vi "Add Hardware.vi"(8 "error in (no error)":errorcluster, 10 "Hardware.lvclass":refnum<class "Hardware.lvclass">, 11 "Controller in":refnum<class "Controller.lvclass">) -> (0 "error out":errorcluster, 3 "Controller out":refnum<class "Controller.lvclass">)   [LabVIEW 2026, in "Controller Actor.lvlib" / "Controller.lvclass"]
uses:
  Controller.lvclass
  C:/Program Files/National Instruments/LabVIEW 2026/vi.lib/ActorFramework/Actor/Actor.lvclass
  Hardware/Hardware.lvclass
  Controller.lvclass/Controller.ctl
  Hardware/Hardware.lvclass/Hardware.ctl
  Extensible-Config-Dialog/Configuration.lvclass/Configuration.ctl
  <vilib>/ActorFramework/Actor/Actor.lvclass/Actor.ctl
  <vilib>/ActorFramework/Message Enqueuer/Message Enqueuer.lvclass/Message Enqueuer.ctl
  <vilib>/ActorFramework/Message Enqueuer/Init from Existing Queue.vi
  Hardware/HW Config/HW Configuration.lvclass
  C:/Users/E2013170/Documents/GitHub/Measurement-Utility-Reference/components/Extensible-Config-Dialog/Configuration.lvclass
  <vilib>/Utility/LVClass/Get LV Class Path.vi
  recovery/packages/oglib_file-4.0.1.22-8A89CE420A/File Group 0/user.lib/_OpenG.lib/file/file.llb/Strip Path Extension__ogtk.vi
  recovery/packages/oglib_file-4.0.1.22-8A89CE420A/File Group 0/user.lib/_OpenG.lib/file/file.llb/Strip Path Extension - String__ogtk.vi
  Extensible-Config-Dialog/Configuration.lvclass
  <vilib>/ActorFramework/Message Enqueuer/Message Enqueuer.lvclass
  Messages/Log Status/Log Status.lvclass
  <vilib>/ActorFramework/Actor/Actor.lvclass
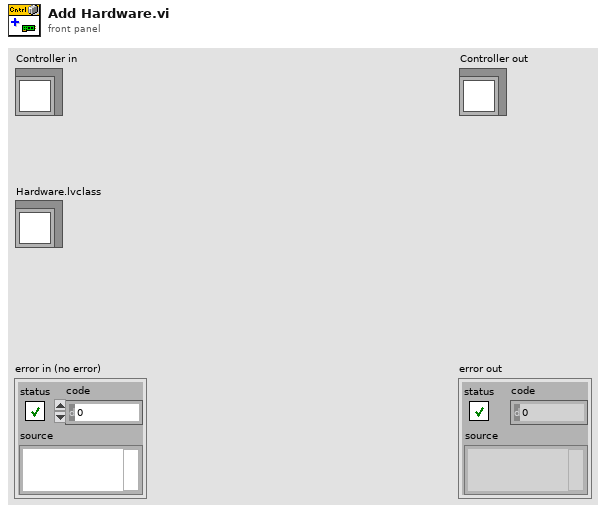
[diagram p1: front panel]
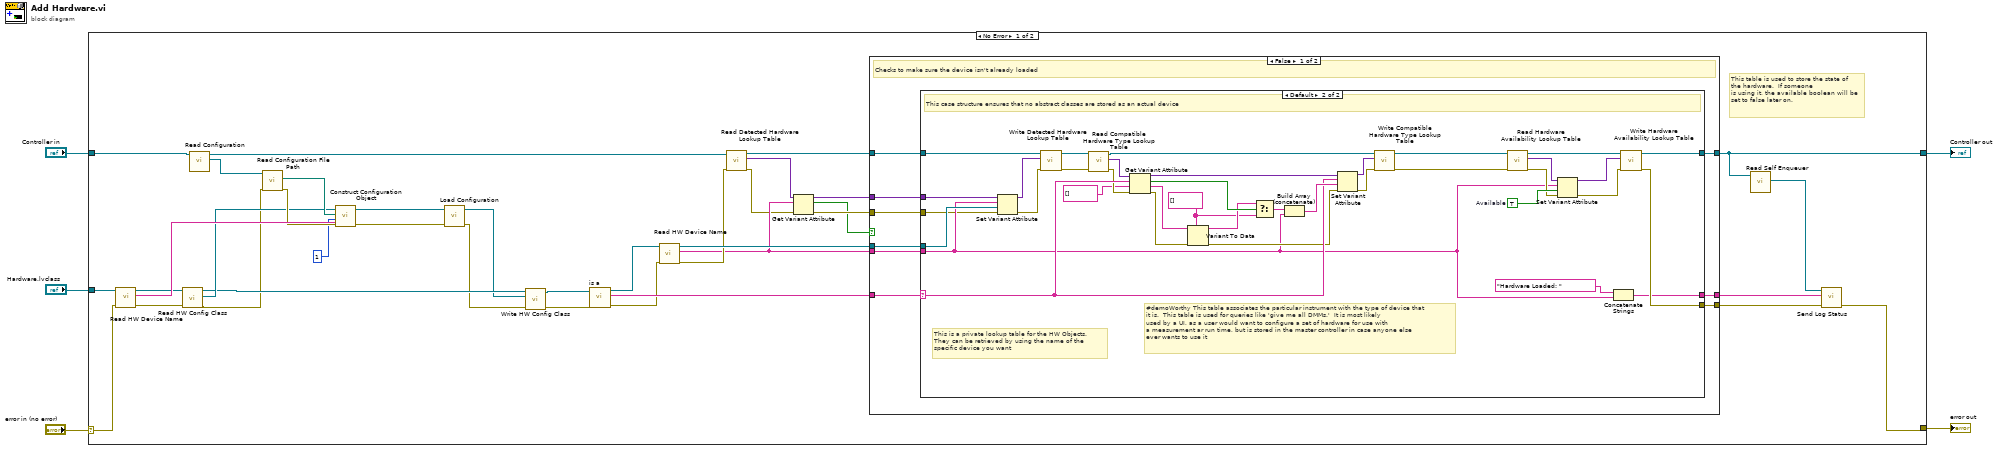
[diagram p0: block diagram]
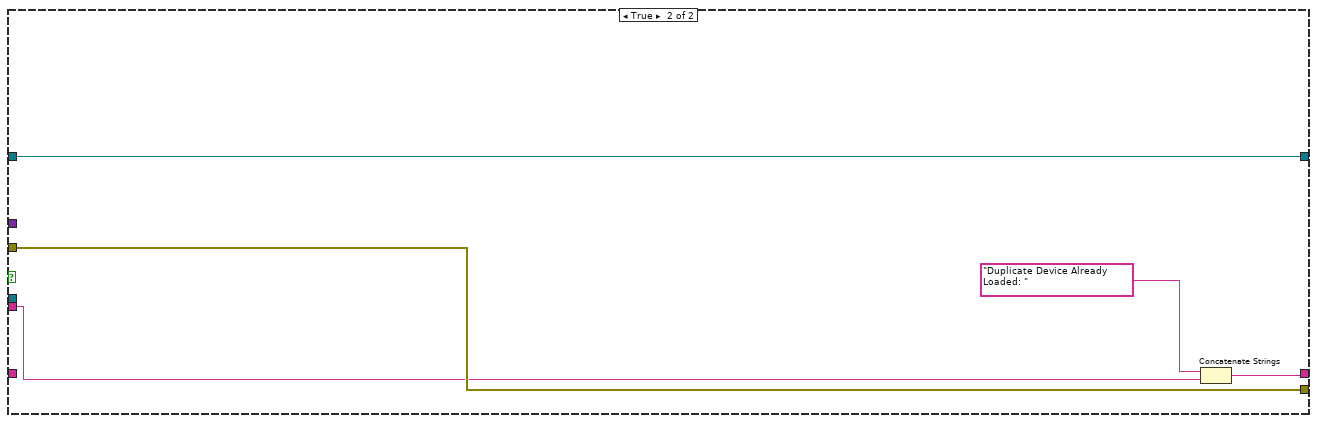
[diagram p3: hidden frame]
diagram:
  n1 = case shown="No Error" "error in (no error)" {
    selector: "error in (no error)" -> [w17 w96]
    tunnel: [w40 w96] -> w4
    tunnel: [w28 w95] -> w2
    tunnel: "Controller in" -> [w21 w95]
    tunnel: "Hardware.lvclass" -> [w19 _]
    frame No Error {
      # "This table is used to store the state of the hardware.  If someone\nis using it, the available boolean will be set to false later on."
      n2 = call "Read HW Device Name.vi"("error in (no error)"=w17, "Analog in"=w19) -> ("error out"=w13:errorcluster, "Device Name"=w18:string, "Analog out"=w14:refnum<class "Hardware.lvclass">)  [unwired: 7 in]
      n3 = call "Read HW Config Class.vi"("error in (no error)"=w13, "Hardware in"=w14) -> ("error out"=w6:errorcluster, "Hardware.lvlib:HW Configuration.lvclass"=w12:refnum<class "HW Configuration.lvclass">, "Hardware out"=w11:refnum<class "Hardware.lvclass">)  [unwired: 7 in]
      n4 = call "Read Configuration.vi"("Controller in"=w21) -> ("Configuration.lvlib:Configuration.lvclass"=w23:refnum<class "Configuration.lvclass">, "Controller out"=w20:refnum<class "Controller.lvclass">)  [unwired: 8 in, 1 out]
      n5 = call "Read Configuration File Path.vi"("error in (no error)"=w6, "Configuration in"=w23) -> ("error out"=w16:errorcluster, "Configuration File Path"=w22:path)  [unwired: 7 in, 1 out]
      n6 = call "Construct Configuration Object.vi"("Group Name"=w18, "error in (no error)"=w16, "Initial Category Selection"=1, "Configuration File Path"=w22, "Configuration in"=w12) -> ("error out"=w24:errorcluster, "Configuration out"=w25:refnum<class "HW Configuration.lvclass">)  [unwired: 3 in, 2 out]
      n7 = call "Load Configuration.vi"("error in (no error)"=w24, "Configuration in"=w25) -> ("error out"=w7:errorcluster, "Configuration out"=w8:refnum<class "HW Configuration.lvclass">)  [unwired: 7 in, 1 out]
      n8 = call "Write HW Config Class.vi"("error in (no error)"=w7, "Hardware.lvlib:HW Configuration.lvclass"=w8, "Hardware in"=w11) -> ("error out"=w9:errorcluster, "Hardware out"=w10:refnum<class "Hardware.lvclass">)  [unwired: 7 in]
      n9 = call-dynamic "is a.vi"("error in (no error)"=w9, "Hardware in"=w10) -> ("error out"=w37:errorcluster, "is a"=w41:string, "Hardware out"=w38:refnum<class "Hardware.lvclass">)  [unwired: 7 in]
      n10 = call "Read HW Device Name.vi"("error in (no error)"=w37, "Analog in"=w38) -> ("error out"=w35:errorcluster, "Device Name"=w32:string, "Analog out"=w39:refnum<class "Hardware.lvclass">)  [unwired: 7 in]
      n11 = call "Read Detected Hardware Lookup Table.vi"("error in (no error)"=w35, "Controller in"=w20) -> ("error out"=w31:errorcluster, "Detected Hardware Lookup Table"=w34:variant, "Controller out"=w36:refnum<class "Controller.lvclass">)  [unwired: 7 in]
      n12 = Get Variant Attribute(Variant=w34, name=w32, error in=w31) -> (duplicate Variant=w33:variant, found=w26:bool, error out=w30:errorcluster)  [unwired: 1 in, 1 out]
      n13 = case shown="False" w26 {
        tunnel: w41 -> [w50 _]
        tunnel: [w49 w93] -> w40
        tunnel: w39 -> [w48 _]
        tunnel: w36 -> [w47 w94]
        tunnel: w33 -> [w46 _]
        tunnel: w32 -> [w45 w90]
        tunnel: w30 -> [w44 w93]
        tunnel: [w43 w94] -> w28
        tunnel: [w42 w91] -> w27
        frame False {
          # "Checks to make sure the device isn't already loaded"
          n14 = case shown="Default" w50 {
            selector: w50 -> [_ w71]
            tunnel: w47 -> [w52 w57]
            tunnel: [w52 w72] -> w43
            tunnel: [w51 w54] -> w49
            tunnel: w48 -> [_ w59]
            tunnel: w45 -> [_ w58]
            tunnel: w46 -> [_ w56]
            tunnel: w44 -> [w51 w55]
            tunnel: [_ w53] -> w42
            frame "Abstract Class" {
            }
            frame Default {
              w77 = TRUE  # Available
              w83 = string[] []
              # "This is a private lookup table for the HW Objects.  \nThey can be retrieved by using the name of the\nspecific device you want"
              # "#demoWorthy This table associates the particular instrument with the type of device that\nit is.  This table is used for queries like 'give me all DMMs.'  It is most likely\nused by a UI, as a user would want to configure a set of hardware for use with\na measurement ar run time, but is stored in the master controller in case anyone else\never wants to use it"
              # "This case structure ensures that no abstract classes are stored as an actual device"
              n15 = Set Variant Attribute(Variant=w56, name=w58, value=w59, error in=w55) -> (Variant out=w89:variant, error out=w68:errorcluster)  [unwired: 1 out]
              n16 = call "Write Detected Hardware Lookup Table.vi"("error in (no error)"=w68, "Detected Hardware Lookup Table"=w89, "Controller in"=w57) -> ("error out"=w69:errorcluster, "Controller out"=w81:refnum<class "Controller.lvclass">)  [unwired: 7 in]
              n17 = call "Read Compatible Hardware Type Lookup Table.vi"("error in (no error)"=w69, "Controller in"=w81) -> ("error out"=w70:errorcluster, "Compatible Hardware Type Lookup Table"=w78:variant, "Controller out"=w80:refnum<class "Controller.lvclass">)  [unwired: 7 in]
              n18 = Get Variant Attribute(Variant=w78, name=w71, default value (empty Variant)=string[] [], error in=w70) -> (duplicate Variant=w82:variant, found=w86:bool, value=w88:string[], error out=w67:errorcluster)
              n19 = Variant To Data(error in=w67, type=w83, Variant=w88) -> (data=w84:string[], error out=w66:errorcluster)
              n20 = Select(t=w84, s=w86, f=w83) -> (s? t:f=w85:string[])
              n21 = Build Array (concatenate)(w85, w58) -> (w87:string[])
              n22 = Set Variant Attribute(Variant=w82, name=w71, value=w87, error in=w66) -> (Variant out=w79:variant, error out=w65:errorcluster)  [unwired: 1 out]
              n23 = call "Write Compatible Hardware Type Lookup Table.vi"("error in (no error)"=w65, "Compatible Hardware Type Lookup Table"=w79, "Controller in"=w80) -> ("error out"=w64:errorcluster, "Controller out"=w76:refnum<class "Controller.lvclass">)  [unwired: 7 in]
              n24 = call "Read Hardware Availability Lookup Table.vi"("error in (no error)"=w64, "Controller in"=w76) -> ("error out"=w63:errorcluster, "Hardware Availability Lookup Table"=w75:variant, "Controller out"=w73:refnum<class "Controller.lvclass">)  [unwired: 7 in]
              n25 = Set Variant Attribute(Variant=w75, name=w58, value=w77, error in=w63) -> (Variant out=w74:variant, error out=w62:errorcluster)  [unwired: 1 out]
              n26 = Concatenate Strings("Hardware Loaded: " ("string"), w58) -> (w53:string)
              n27 = call "Write Hardware Availability Lookup Table.vi"("error in (no error)"=w62, "Hardware Availability Lookup Table"=w74, "Controller in"=w73) -> ("error out"=w54:errorcluster, "Controller out"=w72:refnum<class "Controller.lvclass">)  [unwired: 7 in]
            }
          }
        }
        frame True {
          n28 = Concatenate Strings("Duplicate Device Already Loaded: " ("string"), w90) -> (w91:string)
        }
      }
      n29 = call <vilib>:"Read Self Enqueuer.vi"("Actor"=w28) -> ("Self Enqueuer"=w29:refnum<class "Message Enqueuer.lvclass">)  [unwired: 10 in]
      n30 = call "Send Log Status.vi"("String"=w27, "Message Enqueuer in"=w29) -> ()  [unwired: 8 in, 2 out]
    }
    frame Error {
    }
  }
  "error out" <- w4
  "Controller out" <- w2
